vi "FestoCPX.Station.ProdSuctionGripper.Restore.vi"(8 "error in":errorcluster, 10 "States before clear":bool[](array[boolean])) -> (0 "error out":errorcluster)   [LabVIEW 2016]
uses:
  FestoCPX.DO.Signal.ctl
  Station/Station.ProductSuctionGripper.Type.ctl
  Station/Station.ValvePosition.ctl
  FestoCPX.DO.Data.States.Set.vi
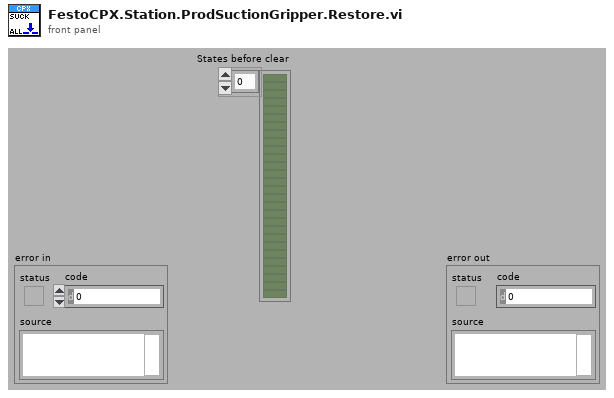
[diagram p1: front panel]
types:
  T1 = typedef "Station.ValvePosition.ctl" = enum16{"Home", "Work"}
  T2 = typedef "Station.ProductSuctionGripper.Type.ctl" = enum8{"Final A", "Final B", "Slot 1 A", "Slot 1 B", "Slot 2 A", "Slot 2 B", "Slot 3 A", "Slot 3 B", "Slot 4 A", "Slot 4 B"}
  T3 = typedef "FestoCPX.DO.Signal.ctl" = enum16{"Safety Reset", "Air Main Valve", "Door Lock", "Button LED Start", "Button LED Stop", "Button LED Control", "Traffic LED Red", "Traffic LED Orange", "Traffic LED Green", "Horn", "Laser Interlock", "Laser Trigger", "Laser Fume Extractor", "Product Suction Gripper Slot 1 A", "Product Suction Gripper Slot 1 B", "Product Suction Gripper Slot 2 A", "Product Suction Gripper Slot 2 B", "Product Suction Gripper Slot 3 A", "Product Suction Gripper Slot 3 B", "Product Suction Gripper Slot 4 A", "Product Suction Gripper Slot 4 B", "Product Suction Gripper Final A", "Product Suction Gripper Final B", "Lamp", "Q1 Product Move Work", "Q1 Product Move Home", "Q2 Table Turn Work", "Q2 Table Turn Home", "Q3 Product Lift A", "Q3 Product Lift B", "Q4 Product Arm OK", "Q4 Product Arm NOK", "Q5 Product Arm Work", "Q6 Product BlowOut A", "Q6 Product BlowOut B"}
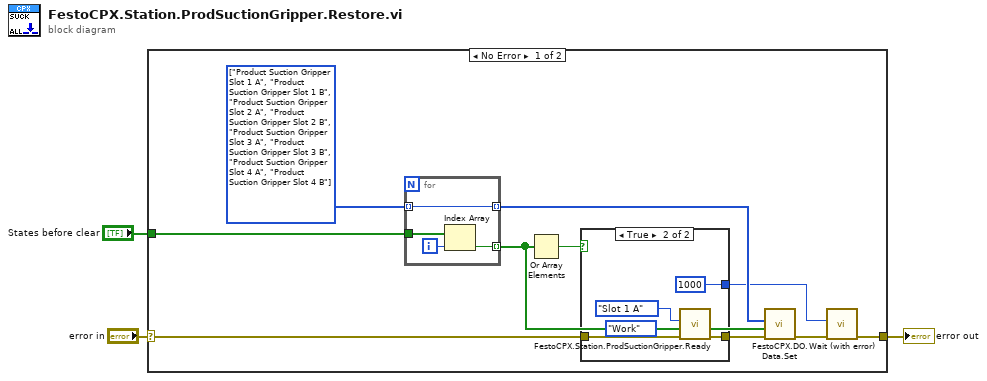
[diagram p0: block diagram]
diagram:
  n1 = case shown="No Error" "error in" {
    selector: "error in" -> [w7 w24]
    tunnel: [w12 w24] -> w3
    tunnel: "States before clear" -> [w11 _]
    frame No Error {
      w10 = T3[] [enum."Product Suction Gripper Slot 1 A", enum."Product Suction Gripper Slot 1 B", enum."Product Suction Gripper Slot 2 A", enum."Product Suction Gripper Slot 2 B", enum."Product Suction Gripper Slot 3 A", enum."Product Suction Gripper Slot 3 B", enum."Product Suction Gripper Slot 4 A", enum."Product Suction Gripper Slot 4 B"] items=["Safety Reset", "Air Main Valve", "Door Lock", "Button LED Start", "Button LED Stop", "Button LED Control", "Traffic LED Red", "Traffic LED Orange", "Traffic LED Green", "Horn", "Laser Interlock", "Laser Trigger", "Laser Fume Extractor", "Product Suction Gripper Slot 1 A", "Product Suction Gripper Slot 1 B", "Product Suction Gripper Slot 2 A", "Product Suction Gripper Slot 2 B", "Product Suction Gripper Slot 3 A", "Product Suction Gripper Slot 3 B", "Product Suction Gripper Slot 4 A", "Product Suction Gripper Slot 4 B", "Product Suction Gripper Final A", "Product Suction Gripper Final B", "Lamp", "Q1 Product Move Work", "Q1 Product Move Home", "Q2 Table Turn Work", "Q2 Table Turn Home", "Q3 Product Lift A", "Q3 Product Lift B", "Q4 Product Arm OK", "Q4 Product Arm NOK", "Q5 Product Arm Work", "Q6 Product BlowOut A", "Q6 Product BlowOut B"] ("CPX.DO")
      n2 = for {
        tunnel: w10 -> [w21] mode=indexing
        tunnel: w11 -> [w23]
        tunnel: [w21] -> w9 mode=indexing
        tunnel: [w20] -> w8 mode=indexing
        i -> [w22]
        n3 = Index Array(array=w23, index=w22) -> (element=w20:bool)
      }
      n4 = Or Array Elements(Boolean array=w8) -> (logical OR=w5:bool)
      n5 = case shown="True" w5 {
        tunnel: w7 -> [w14 w19]
        tunnel: [w14 w18] -> w6
        tunnel: [_ u32 1000 ("milliseconds to wait")] -> w4
        frame False {
        }
        frame True {
          n6 = call "FestoCPX.Station.ProdSuctionGripper.Ready.vi"("error in"=w19, "Position"=Station.ValvePosition."Work", "Type"=Station.ProductSuctionGripper.Type."Slot 1 A") -> ("error out"=w18:errorcluster)  [unwired: 7 in, 1 out]
        }
      }
      n7 = call-poly "FestoCPX.DO.Data.Set.vi"("error in (no error)"=w6, "State"=w8, "CPX.DO"=w9) -> ("error out"=w13:errorcluster)  [unwired: 8 in]
      n8 = call "Wait (with error).vi"("error in (no error)"=w13, "milliseconds to wait"=w4) -> ("error out"=w12:errorcluster)  [unwired: 8 in, 1 out]
    }
    frame Error {
    }
  }
  "error out" <- w3
